vi "Global 1.vi"() -> ()   [LabVIEW 2012]
panel:
  out "Moving?":bool
  out "Homed?":bool
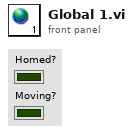
[diagram p1: front panel]
diagram:
